vi "1D Buffer UI.vi"(0 "Data In":T4 {"time" format="%<%H:%M:%S%2u>T"}, 2 "Display State In":T2 {"Time" format="%<%H:%M:%S>T"}, 3 "Container State":T3) -> (6 "Data Out":T4 {"time" format="%<%H:%M:%S%2u>T"}, 7 "Display State Out":T2 {"Time" format="%<%H:%M:%S>T"}, 8 "Action":T1)   [LabVIEW 2015, in "1D Xctl Buffer.xctl"]
uses:
  1D Xctl Buffer.xctl
  1D Buffer Data.ctl
  <vilib>/_xctls/Container State.ctl
  1D Buffer State.ctl
  <vilib>/_xctls/Action.ctl
  <vilib>/_xctls/XControlSupport.lvlib
panel:
  out "1D Graph":cluster{"Time":timestamp[], u16[]}(graph)
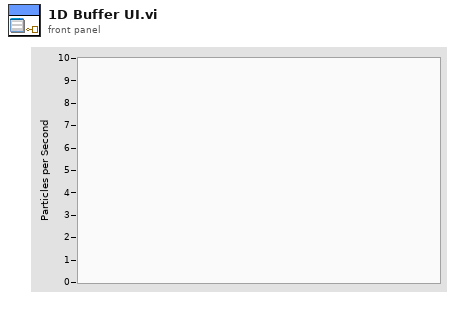
[diagram p1: front panel]
types:
  T1 = typedef "XControlSupport.lvlib/Action.ctl" = cluster{"Data Changed?":bool, "State Changed?":bool, "Action Name":string}
  T2 = typedef "1D Xctl Buffer.xctl/1D Buffer State.ctl" = cluster{"History":i32, "Time":timestamp[], "Data":u16[]}
  T3 = typedef "XControlSupport.lvlib/Container State.ctl" = cluster{"Indicator?":bool, "Run Mode?":bool, " Refnum":refnum<vi>}
  T4 = typedef "1D Xctl Buffer.xctl/1D Buffer Data.ctl" = cluster{"time":timestamp, "val":u16}
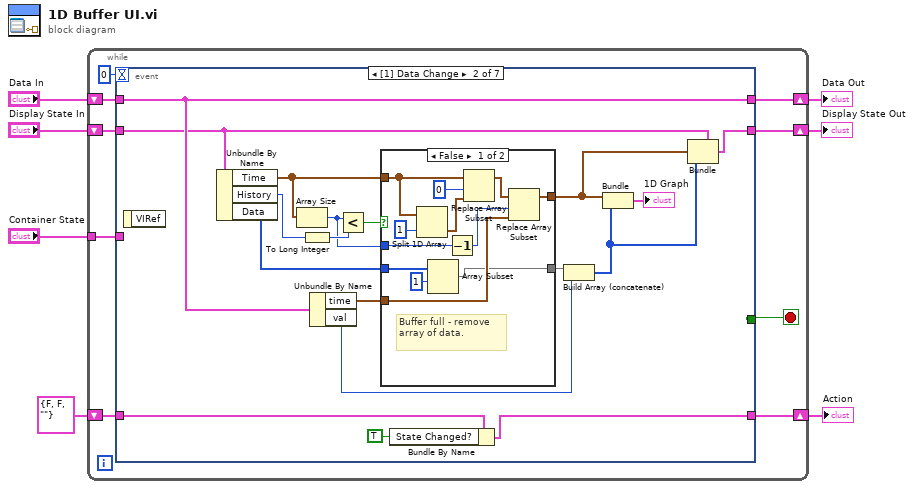
[diagram p0: block diagram]
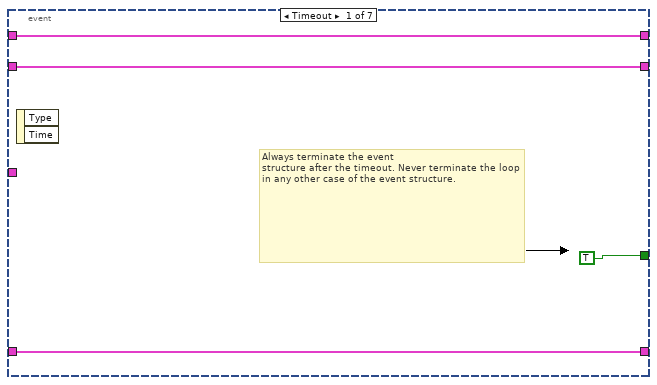
[diagram p2: hidden frame]
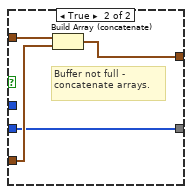
[diagram p3: hidden frame]
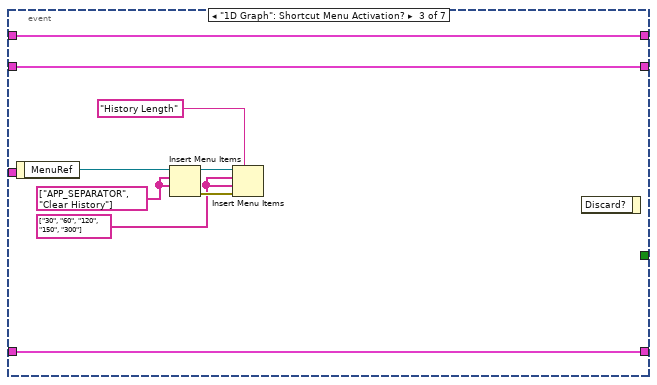
[diagram p4: hidden frame]
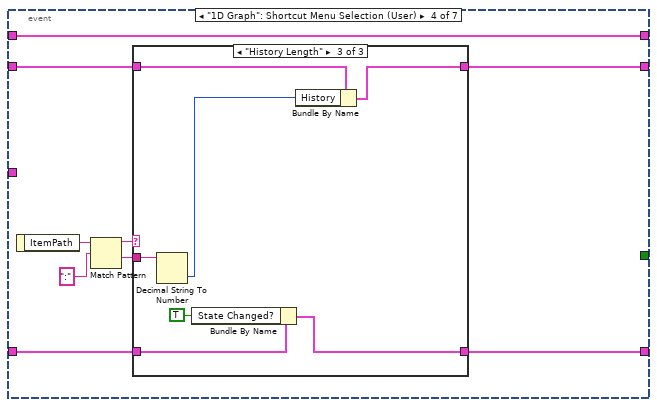
[diagram p5: hidden frame]
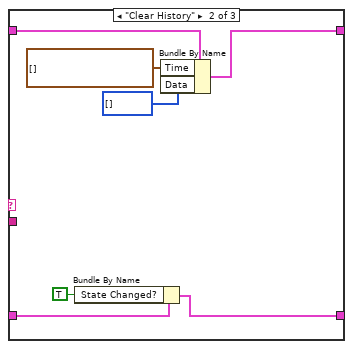
[diagram p7: hidden frame]
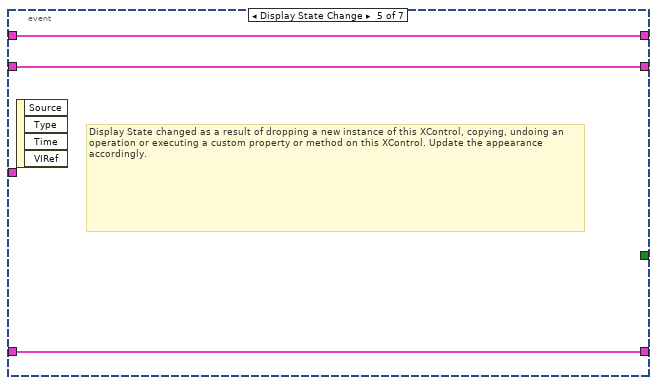
[diagram p8: hidden frame]
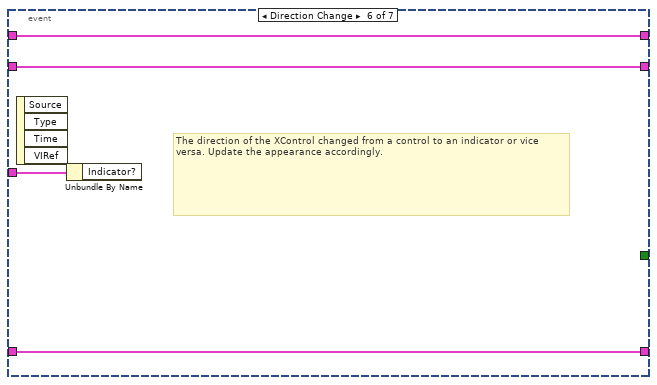
[diagram p9: hidden frame]
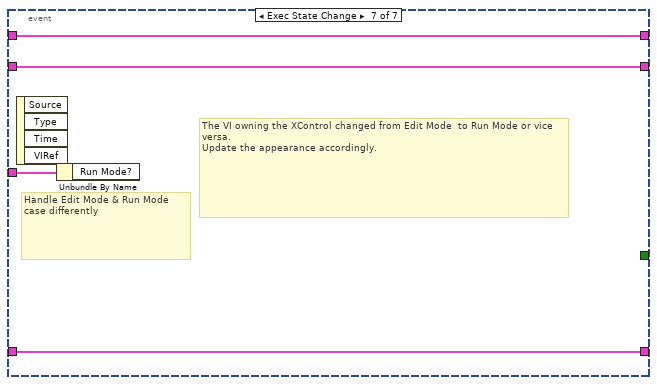
[diagram p10: hidden frame]
diagram:
  n1 = while {
    shift-right: [w15] -> w4
    shift-left: "Display State In" -> [w16]
    tunnel: "Container State" -> [w12]
    shift-right: [w10] -> w7
    shift-left: "Data In" -> [w11]
    shift-right: [w8] -> w2
    shift-left: T1 {"Data Changed?"=FALSE, "State Changed?"=FALSE, "Action Name"=""} ("Action") -> [w9]
    stop <- w14 stop-if-true
    n2 = event shown="[1] Data Change" {
      selector: _ -> [_ _ _ _ _ _ _]
      dyn-events: _ -> [_ _ _ _ _ _ _]
      timeout: 0 -> [_ _ _ _ _ _ _]
      tunnel: w16 -> [w18 w24 w63 w69 w91 w94 w98]
      tunnel: [w18 w21 w63 w68 w91 w94 w98] -> w15
      tunnel: [TRUE _ _ _ _ _ _] -> w14
      tunnel: w12 -> [_ _ _ _ _ w95 w99]
      tunnel: w11 -> [w17 w38 w62 w72 w90 w93 w97]
      tunnel: [w17 w38 w62 w72 w90 w93 w97] -> w10
      tunnel: [w19 w26 w61 w70 w89 w92 w96] -> w8
      tunnel: w9 -> [w19 w27 w61 w71 w89 w92 w96]
      event Timeout {
        # "Always terminate the event\nstructure after the timeout. Never terminate the loop in any other case of the event structure."
        n3 = event-data() -> ()  [unwired: 1 in, 2 out]
      }
      event Data Change {
        n4 = event-data() -> ()  [unwired: 1 in, 1 out]
        n5 = Unbundle By Name(w24) -> ("Time"=w34:timestamp[], "History"=w33:i32, "Data"=w36:u16[])
        n6 = Array Size(array=w34) -> (size(s)=w31:i32)
        n7 = To Long Integer(number=w33) -> (32bit integer=w35:i32)
        n8 = Unbundle By Name(w38) -> ("time"=w37:timestamp, "val"=w29:u16)
        n9 = Less?(x=w31, y=w35) -> (x < y?=w32:bool)
        n10 = case shown="False" w32 {
          tunnel: w34 -> [w45 w54]
          tunnel: [w44 w52] -> w23
          tunnel: w37 -> [w43 w53]
          tunnel: w36 -> [w40 w51]
          tunnel: w31 -> [w42 _]
          tunnel: [w39 w51] -> w30
          frame False {
            # "Buffer full - remove array of data."
            n11 = Split 1D Array(array=w45, index=1) -> (second subarray=w46:timestamp[])  [unwired: 1 out]
            n12 = Array Subset(array=w40, index=1) -> (w39:u16[])  [unwired: 1 in]
            n13 = Decrement(x=w42) -> (x-1=w48:i32)
            n14 = Replace Array Subset(array=w45, new element=w46, index=0) -> (w49:timestamp[])
            n15 = Replace Array Subset(array=w49, new element=w43, index=w48) -> (w44:timestamp[])
          }
          frame True {
            # "Buffer not full - concatenate arrays."
            n16 = Build Array (concatenate)(w54, w53) -> (w52:timestamp[])
          }
        }
        n17 = Bundle By Name(cluster=w27, "State Changed?"=TRUE) -> (w26:T1)
        n18 = Build Array (concatenate)(w30, w29) -> (w22:u16[])
        n19 = Bundle("Time"=w23, w22) -> (→"1D Graph":cluster{"Time":timestamp[], u16[]})  [unwired: 1 in]
        n20 = Bundle(cluster=w24, "Time"=w23, "Data"=w22) -> (w21:T2)  [unwired: 1 in]
      }
      event "1D Graph": Shortcut Menu Activation? {
        w55 = string[] ["30", "60", "120", "150", "300"] ("item names")
        w59 = string[] ["APP_SEPARATOR", "Clear History"]
        n21 = event-data() -> ("MenuRef"=w60:refnum<k9>)  [unwired: 1 in]
        n22 = Insert Menu Items(7:w59, 8:w59, 9:w60) -> (0:w57:errorcluster, 3:w58:refnum<k9>)  [unwired: 3 in, 1 out]
        n23 = Insert Menu Items(5:"History Length" ("menu tag"), 6:w57, 7:w55, 8:w55, 9:w58) -> ()  [unwired: 1 in, 3 out]
        n24 = event-data() -> ()  [unwired: 2 in, 1 out]
      }
      event "1D Graph": Shortcut Menu Selection (User) {
        n25 = event-data() -> ("ItemPath"=w67:string)  [unwired: 1 in]
        n26 = Match Pattern(string=w67, regular expression=":") -> (before substring=w65:string, after substring=w64:string)  [unwired: 1 in, 2 out]
        n27 = case shown="\"History Length\"" w65 {
          tunnel: w71 -> [w74 w81 w84]
          tunnel: [w74 w79 w83] -> w70
          tunnel: w69 -> [w73 w78 w87]
          tunnel: [w73 w75 w86] -> w68
          tunnel: w64 -> [_ _ w88]
          frame "False", Default {
          }
          frame "Clear History" {
            n28 = Bundle By Name(cluster=w81, "State Changed?"=TRUE) -> (w79:T1)
            n29 = Bundle By Name(cluster=w78, "Time"=timestamp[] [], "Data"=u16[] []) -> (w75:T2)
          }
          frame "History Length" {
            n30 = Decimal String To Number(string=w88) -> (number=w85:i32)  [unwired: 2 in, 1 out]
            n31 = Bundle By Name(cluster=w84, "State Changed?"=TRUE) -> (w83:T1)
            n32 = Bundle By Name(cluster=w87, "History"=w85) -> (w86:T2)
          }
        }
      }
      event Display State Change {
        # "Display State changed as a result of dropping a new instance of this XControl, copying, undoing an operation or executing a custom property or method on this XControl. Update the appearance accordingly."
        n33 = event-data() -> ()  [unwired: 1 in, 4 out]
      }
      event Direction Change {
        # "The direction of the XControl changed from a control to an indicator or vice versa. Update the appearance accordingly."
        n34 = event-data() -> ()  [unwired: 1 in, 4 out]
        n35 = Unbundle By Name(w95) -> ()  [unwired: 1 out]
      }
      event Exec State Change {
        # "The VI owning the XControl changed from Edit Mode  to Run Mode or vice versa.\nUpdate the appearance accordingly."
        # "Handle Edit Mode & Run Mode\ncase differently"
        n36 = event-data() -> ()  [unwired: 1 in, 4 out]
        n37 = Unbundle By Name(w99) -> ()  [unwired: 1 out]
      }
    }
  }
  "Display State Out" <- w4
  "Data Out" <- w7
  "Action" <- w2
